vi "ReplaceConstantNode.vi"(5 "Old Control Name":string, 7 "New Control Name":string, 8 "error in (no error)":errorcluster, 11 "VI Refnum In":refnum<vi>) -> (0 "error out":errorcluster, 3 "VI Refnum Out":refnum<vi>, 4 "Replaced":bool)   [LabVIEW 2024]
uses:
  <vilib>/Utility/traverseref.llb/TRef TravTarget.ctl
  <vilib>/Utility/traverseref.llb/VI Scripting - Traverse.lvlib
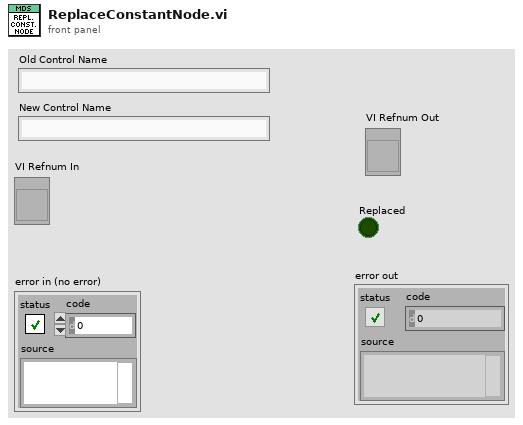
[diagram p1: front panel]
types:
  T1 = typedef "TRef TravTarget.ctl" = enum16{"FP", "BD", "Other"}
  T2 = enum32{"not a typedef", "typedef", "strict typedef", "class private data"}
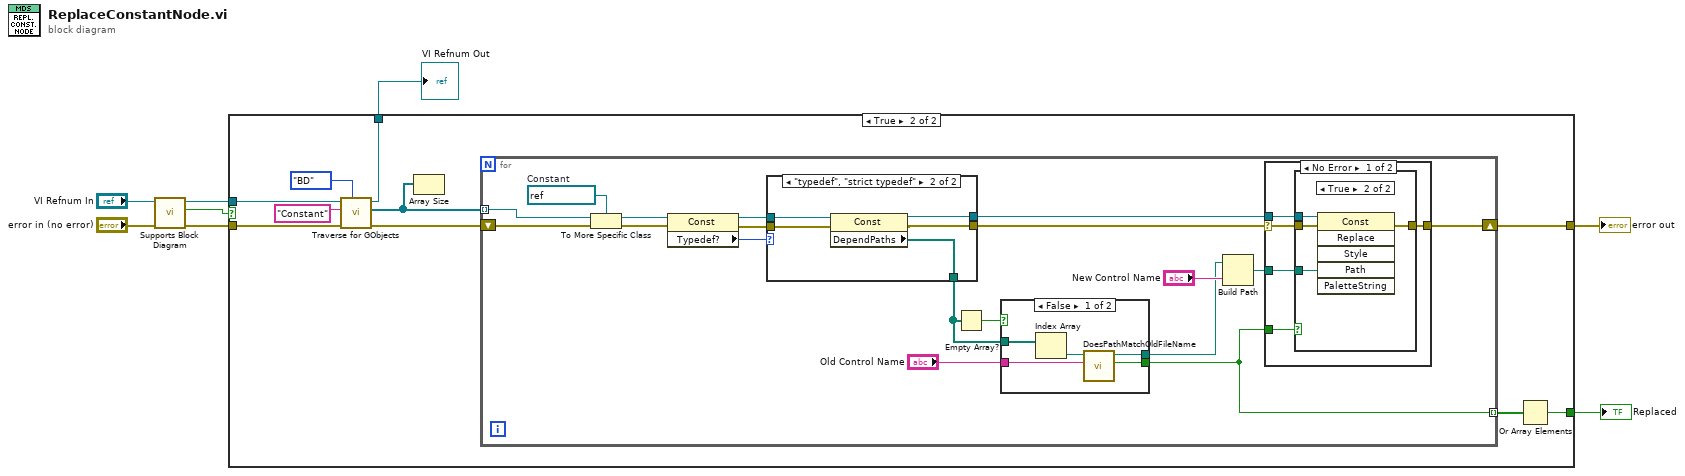
[diagram p0: block diagram]
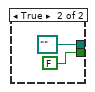
[diagram p3: hidden frame]
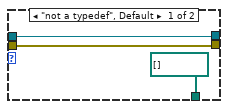
[diagram p4: hidden frame]
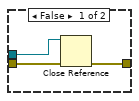
[diagram p5: hidden frame]
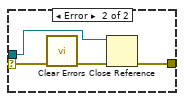
[diagram p6: hidden frame]
diagram:
  n1 = call "Supports Block Diagram.vi"("error in (no error)"="error in (no error)", "vi in"="VI Refnum In") -> ("error out"=w2:errorcluster, "has block diagram"=w1:bool, "vi out"=w3:refnum<vi>)  [unwired: 7 in]
  n2 = case shown="True" w1 {
    tunnel: [_ w11] -> w8
    tunnel: w2 -> [w9 w17]
    tunnel: w3 -> [w10 w16]
    tunnel: [w9 w14] -> w7
    tunnel: [w10 w13] -> w6
    frame False {
    }
    frame True {
      n3 = call <vilib>:"Traverse for GObjects.vi"("Traverse Target"=TRef_TravTarget."BD", "error in (no error)"=w17, "Class Name"="Constant", "VI Refnum"=w16) -> ("error out"=w20:errorcluster, "References"=w15:refnum<vi>[], "dup VI Refnum"=w13:refnum<vi>)  [unwired: 4 in, 1 out]
      n4 = Array Size(array=w15) -> ()  [unwired: 1 out]
      n5 = for {
        shift-right: [w36] -> w14
        shift-left: w20 -> [w37]
        tunnel: w15 -> [w38] mode=indexing
        tunnel: [w24] -> w12 mode=indexing
        w33 = refnum<vi> refnum  # Constant
        n6 = To More Specific Class(target class=w33, reference=w38, error in=w37) -> (specific class reference=w32:refnum<vi>, error out=w31:errorcluster)
        n7 = property class="Const"(reference=w32, error in=w31) -> (reference out=w28:refnum<vi>, error out=w30:errorcluster, "Typedef?"=w26:T2)
        n8 = case shown="\"typedef\", \"strict typedef\"" w26 {
          tunnel: [path[] [] ("MissingPaths") w53] -> w21
          tunnel: w30 -> [w46 w52]
          tunnel: [w46 w51] -> w29
          tunnel: w28 -> [w47 w50]
          tunnel: [w47 w49] -> w27
          frame "not a typedef", Default {
          }
          frame "typedef", "strict typedef" {
            n9 = property class="Const"(reference=w50, error in=w52) -> (reference out=w49:refnum<vi>, error out=w51:errorcluster, "DependPaths"=w53:path[])
          }
        }
        n10 = Empty Array?(array=w21) -> (empty?=w22:bool)
        n11 = case shown="False" w22 {
          tunnel: "Old Control Name" -> [w42 _]
          tunnel: [w41 FALSE ("Match Found")] -> w24
          tunnel: [w40 path "" ("Parent Directory")] -> w23
          tunnel: w21 -> [w39 _]
          frame False {
            n12 = Index Array(array=w39) -> (element=w43:path)  [unwired: 1 in]
            n13 = call "DoesPathMatchOldFileName.vi"("Old File Name"=w42, "File Path"=w43) -> ("Match Found"=w41:bool, "Parent Directory"=w40:path)  [unwired: 8 in]
          }
          frame True {
          }
        }
        n14 = Build Path(base path=w23, name or relative path="New Control Name") -> (appended path=w35:path)
        n15 = case shown="No Error" w29 {
          selector: w29 -> [w54 w69]
          tunnel: w35 -> [w58 _]
          tunnel: w24 -> [w57 _]
          tunnel: [w56 w67] -> w36
          tunnel: w27 -> [w55 w66]
          frame No Error {
            n16 = case shown="True" w57 {
              tunnel: w58 -> [_ w65]
              tunnel: w54 -> [w61 w64]
              tunnel: [w60 w63] -> w56
              tunnel: w55 -> [w59 w62]
              frame False {
                n17 = Close Reference(reference=w59, error in (no error)=w61) -> (error out=w60:errorcluster)
              }
              frame True {
                n18 = invoke class="Const" method="Replace"(reference=w62, error in=w64, "Path"=w65) -> (error out=w63:errorcluster)  [unwired: 3 in, 5 out]
              }
            }
          }
          frame Error {
            n19 = call <vilib>:"Clear Errors.vi"("error in (no error)"=w69) -> ("error out"=w68:errorcluster)  [unwired: 5 in, 1 out]
            n20 = Close Reference(reference=w66, error in (no error)=w68) -> (error out=w67:errorcluster)
          }
        }
      }
      n21 = Or Array Elements(Boolean array=w12) -> (logical OR=w11:bool)
    }
  }
  "error out" <- w7
  "Replaced" <- w8
  "VI Refnum Out" <- w6
